vi "SV Get By Measurement Type.vi"   [LabVIEW 2017]
doc: "Separates data from an array of waveforms based on the type of measurement selected. This VI requires that waveform attributes such as NI_UnitDescription are added by NI DAQmx."
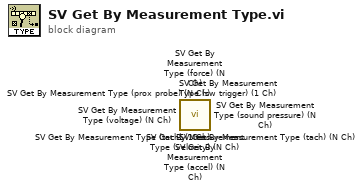
[diagram p0: block diagram]
diagram:
  n1 = call <vilib>:"SV Get By Measurement Type (velocity) (N Ch).vi"() -> ()  [unwired: 13 in, 3 out]
  n2 = call <vilib>:"SV Get By Measurement Type (sw trigger) (1 Ch).vi"() -> ()  [unwired: 9 in, 7 out]
  n3 = call <vilib>:"SV Get By Measurement Type (voltage) (N Ch).vi"() -> ()  [unwired: 13 in, 3 out]
  n4 = call <vilib>:"SV Get By Measurement Type (sound pressure) (N Ch).vi"() -> ()  [unwired: 13 in, 3 out]
  n5 = call <vilib>:"SV Get By Measurement Type (prox probe) (N Ch).vi"() -> ()  [unwired: 11 in, 5 out]
  n6 = call <vilib>:"SV Get By Measurement Type (force) (N Ch).vi"() -> ()  [unwired: 13 in, 3 out]
  n7 = call <vilib>:"SV Get By Measurement Type (accel) (N Ch).vi"() -> ()  [unwired: 13 in, 3 out]
  n8 = call <vilib>:"SV Get By Measurement Type (tach) (N Ch).vi"() -> ()  [unwired: 13 in, 3 out]
  n9 = call <vilib>:"SV Get By Measurement Type (tach) (1 Ch).vi"() -> ()  [unwired: 8 in, 8 out]
